vi "Compute Chirp Parameters-Core.vi"(10 "AOL_Globals":T3={"Imaging Protocol"=enum."AOL Z-Stack", "Number of POI"=0, "Number of Miniscans"=0, "Number of Trials"=0, "Number of Cycles "=0, "# Averaged Frames"=0, "Laser power (%)"=0, "Pockels (V)"=0.0, "Acquisition Length (sec)"=0.0, "Fill time (us)"=0.0, "POI Dwell time (us)"=0.0, "Miniscan Dwell time per pixel (us)"=0.0, "PMT 1"=0.0, "PMT 2"=0.0, "Back Apperture (mA)"=0.0, "Frame Size"=0, "Center Frequency"=0.0, "Field of View (um)"=175.0, "Field of View (norm)"=0.0, "DwellTime (us)"=0.0, "Ref Dwell Time (us)"=0.0, "Wavelength (nm)"=0.0, "Zoom"=0.0, "AOL Z"=0.0, "AOL Mode"=enum."Raster", "GridXY"=0.0, "GridZ"=0.0, "TriggerPeriod (sec)"=0.0, "Number of Pixels in Miniscan"=0, "Experiment folder path"=path "", "X centre"=0.0, "Y centre"=0.0, "Angle (degrees)"=0.0, "Angle Xs (degrees)"=0.0, "Angle Ys (degrees)"=0.0, "Plane Mode"=0, "Threshold"=[], "Regenerate Chirps"=FALSE, "Rectangle ROI length (pixels)"=0, "Rectangle ROI height (pixels)"=0, "AOD fill"=4900, "StartupDelay"=0, "Samples Wait after Trigger"=5080, "Slip Cycle"=600000, "Add Cycle"=TRUE, "Functional Mode"=enum."Point", "Z Start"=0.0, "Z Stop"=0.0, "# Planes"=0, "Total Pixels"=0, "Variable Miniscan Pixels"=[], "Use Variable Length"=FALSE, "Use Variable Resolution"=FALSE, "Laser power (%) at Z Start"=0, "Laser power (%) at Z Stop"=0, "Ref Z Step"=0} {"Angle Ys (degrees)" format="%#.6g"; "Angle Xs (degrees)" format="%#.6g"; "Plane Mode" items=["XY Plane", "XZ Plane", "YZ Plane", "arbitraryplane"]; "Frame Size" items=["100X100"=100, "128X128"=128, "200X200"=200, "256X256"=256, "512X512"=512, "1024x1024"=1024, "2048x2048"=2048]; "Back Apperture (mA)" format="%#.6g"; "Pockels (V)" format="%#.6g"; "PMT 2" format="%#.6g"; "PMT 1" format="%#.6g"; "Angle (degrees)" format="%#.6g"; "POI Dwell time (us)" format="%#.6g"}, 11 "Chirp in":cluster{"HexPackets":string[]}) -> (0 "error out":errorcluster, 1 "Z-stack chirp parameters":cluster{"HexPackets":string[]}[](array[cluster]), 2 "# of Z-planes":i32, 3 "Chirp out":cluster{"HexPackets":string[]})   [LabVIEW 2020]
uses:
  Typedefs/Controls/AOL_Globals.ctl
  Typedefs/Imaging Protocols enum.ctl
  Typedefs/Frame Size.ctl
  Typedefs/AOL modes.ctl
  Typedefs/Plane Mode.ctl
  Typedefs/Functional Mode.ctl
  Typedefs/ROI XY coordinates cluster.ctl
  Typedefs/Chirp_ABCD.ctl
  Typedefs/Read Write Enum.ctl
  Global Variables/General Globals.vi
panel:
  out "Chirp Parameters":T1
  out "ROI Coordinates (broken down to miniscans)":T2
  out "HexPackets":string[](array[string])
  out "AOL_Globals 2":T3={"Imaging Protocol"=enum."Live Imaging", "Number of POI"=0, "Number of Miniscans"=0, "Number of Trials"=0, "Number of Cycles "=0, "# Averaged Frames"=0, "Laser power (%)"=0, "Pockels (V)"=0.0, "Acquisition Length (sec)"=0.0, "Fill time (us)"=0.0, "POI Dwell time (us)"=0.0, "Miniscan Dwell time per pixel (us)"=0.0, "PMT 1"=0.0, "PMT 2"=0.0, "Back Apperture (mA)"=0.0, "Frame Size"=200, "Center Frequency"=0.0, "Field of View (um)"=175.0, "Field of View (norm)"=0.0, "DwellTime (us)"=0.0, "Ref Dwell Time (us)"=0.0, "Wavelength (nm)"=0.0, "Zoom"=0.0, "AOL Z"=0.0, "AOL Mode"=enum."Raster", "GridXY"=0.0, "GridZ"=0.0, "TriggerPeriod (sec)"=0.0, "Number of Pixels in Miniscan"=0, "Experiment folder path"=path "", "X centre"=0.0, "Y centre"=0.0, "Angle (degrees)"=0.0, "Angle Xs (degrees)"=0.0, "Angle Ys (degrees)"=0.0, "Plane Mode"=0, "Threshold"=[], "Regenerate Chirps"=FALSE, "Rectangle ROI length (pixels)"=0, "Rectangle ROI height (pixels)"=0, "AOD fill"=4900, "StartupDelay"=0, "Samples Wait after Trigger"=5080, "Slip Cycle"=600000, "Add Cycle"=TRUE, "Functional Mode"=enum."Point", "Z Start"=0.0, "Z Stop"=0.0, "# Planes"=0, "Total Pixels"=0, "Variable Miniscan Pixels"=[], "Use Variable Length"=FALSE, "Use Variable Resolution"=FALSE, "Laser power (%) at Z Start"=0, "Laser power (%) at Z Stop"=0, "Ref Z Step"=0} {"Angle Ys (degrees)" format="%#.6g"; "Angle Xs (degrees)" format="%#.6g"; "Plane Mode" items=["XY Plane", "XZ Plane", "YZ Plane", "arbitraryplane"]; "Frame Size" items=["100X100"=100, "128X128"=128, "200X200"=200, "256X256"=256, "512X512"=512, "1024x1024"=1024, "2048x2048"=2048]; "Back Apperture (mA)" format="%#.6g"; "Pockels (V)" format="%#.6g"; "PMT 2" format="%#.6g"; "PMT 1" format="%#.6g"; "Angle (degrees)" format="%#.6g"; "POI Dwell time (us)" format="%#.6g"}
  out "?":i32
  out "?":i32
  out "Execution time 2":u32
  out "Execution time":u32
  out "Imaging Protocol":T4
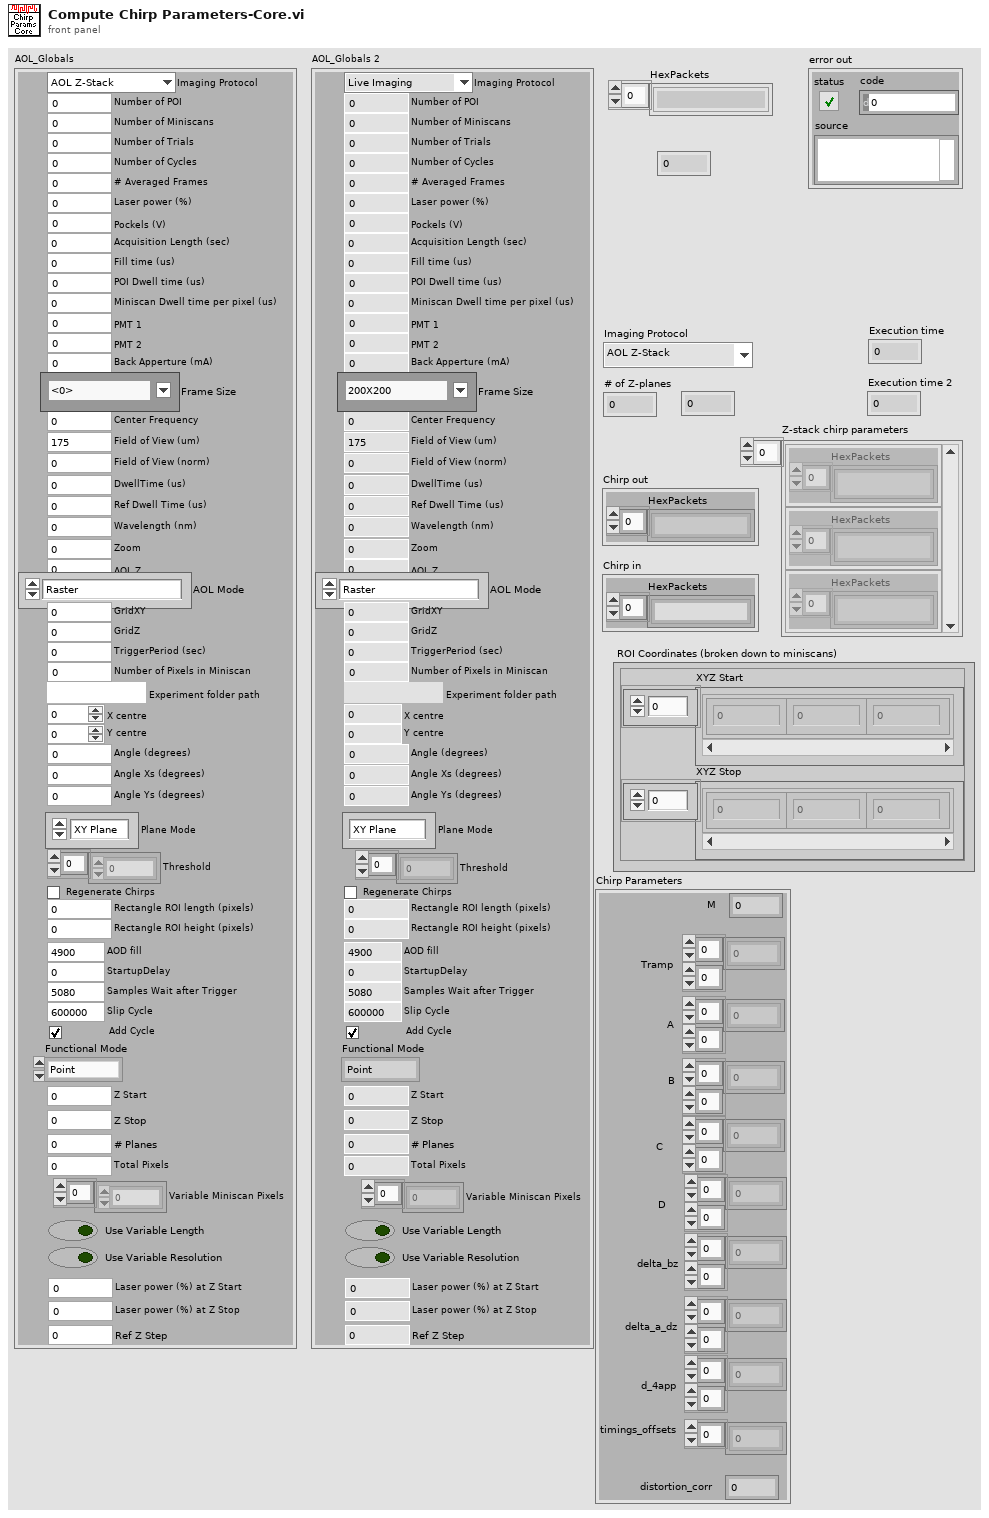
[diagram p1: front panel]
types:
  T1 = typedef "Chirp_ABCD.ctl" = cluster{"M ":dbl, "Tramp":dbl[][], "A":dbl[][], "B":dbl[][], "C":dbl[][], "D":dbl[][], "delta_bz":dbl[][], "delta_a_dz":dbl[][], "d_4app":dbl[][], "timings_offsets":dbl[], "distortion_corr":dbl}
  T2 = typedef "ROI XY coordinates cluster.ctl" = cluster{"XYZ Start":cluster{"X":sgl, "Y":sgl, "Z":sgl}[], "XYZ Stop":cluster{"X":sgl, "Y":sgl, "Z":sgl}[]}
  T3 = typedef "AOL_Globals.ctl" = cluster{"Imaging Protocol":T4, "Number of POI":u16, "Number of Miniscans":u16, "Number of Trials":u16, "Number of Cycles ":u64, "# Averaged Frames":u16, "Laser power (%)":u8, "Pockels (V)":dbl, "Acquisition Length (sec)":dbl, "Fill time (us)":dbl, "POI Dwell time (us)":dbl, "Miniscan Dwell time per pixel (us)":dbl, "PMT 1":dbl, "PMT 2":dbl, "Back Apperture (mA)":dbl, "Frame Size":T5, "Center Frequency":dbl, "Field of View (um)":dbl, "Field of View (norm)":dbl, "DwellTime (us)":dbl, "Ref Dwell Time (us)":dbl, "Wavelength (nm)":dbl, "Zoom":dbl, "AOL Z":dbl, "AOL Mode":T6, "GridXY":dbl, "GridZ":dbl, "TriggerPeriod (sec)":dbl, "Number of Pixels in Miniscan":u16, "Experiment folder path":path, "X centre":dbl, "Y centre":dbl, "Angle (degrees)":dbl, "Angle Xs (degrees)":dbl, "Angle Ys (degrees)":dbl, "Plane Mode":T7, "Threshold":u16[], "Regenerate Chirps":bool, "Rectangle ROI length (pixels)":u16, "Rectangle ROI height (pixels)":u16, "AOD fill":u16, "StartupDelay":i32, "Samples Wait after Trigger":u16, "Slip Cycle":u32, "Add Cycle":bool, "Functional Mode":T8, "Z Start":dbl, "Z Stop":dbl, "# Planes":i32, "Total Pixels":i32, "Variable Miniscan Pixels":u16[], "Use Variable Length":bool, "Use Variable Resolution":bool, "Laser power (%) at Z Start":u8, "Laser power (%) at Z Stop":u8, "Ref Z Step":i8}
  T4 = typedef "Imaging Protocols enum.ctl" = enum16{"AOL Z-Stack", "Motor Z Stack", "Parameter Sweep", "Functional Acquisition", "Single Plane Acquisition", "Volume Acquisition", "Live Imaging", "Live Plane Imaging", "Live Volume Imaging"}
  T5 = typedef "Frame Size.ctl" = u16
  T6 = typedef "AOL modes.ctl" = enum16{"Raster", "Structural", "Pointing", "Mini Scan", "Alignment"}
  T7 = typedef "Plane Mode.ctl" = u16
  T8 = typedef "Functional Mode.ctl" = enum16{"Point", "Line", "Patch", "Plane", "Volume"}
  T9 = typedef "Read Write Enum.ctl" = enum16{"Read", "Write"}
  T10 = cluster{"XYZ Start":cluster{"X":sgl, "Y":sgl, "Z":sgl}[], "XYZ Stop":cluster{"X":sgl, "Y":sgl, "Z":sgl}[]}
  T11 = typedef "ROI parameters data type.ctl" = cluster{"ROI index":dbl, "ROI ID":dbl, "ROI Time (ns)":dbl, "Pixels in ROI":dbl, "X start":dbl, "Y start":dbl, "Z start":dbl, "X stop":dbl, "Y stop":dbl, "Z stop":dbl, "Angle (deg)":dbl, "Composite ID":dbl, "Number of lines":dbl, "Frame Size":dbl, "Zoom":dbl, "Laser Power (%)":dbl, "ROI group ID":dbl, "Resolution":dbl, "Dwell Time per pixel":dbl, "Pixels per miniscan":dbl, "Original FOV (um)":dbl, "Apparent Frame Size":dbl, "Z Plane Idx":i32[], "Z Plane codes":i32[]}
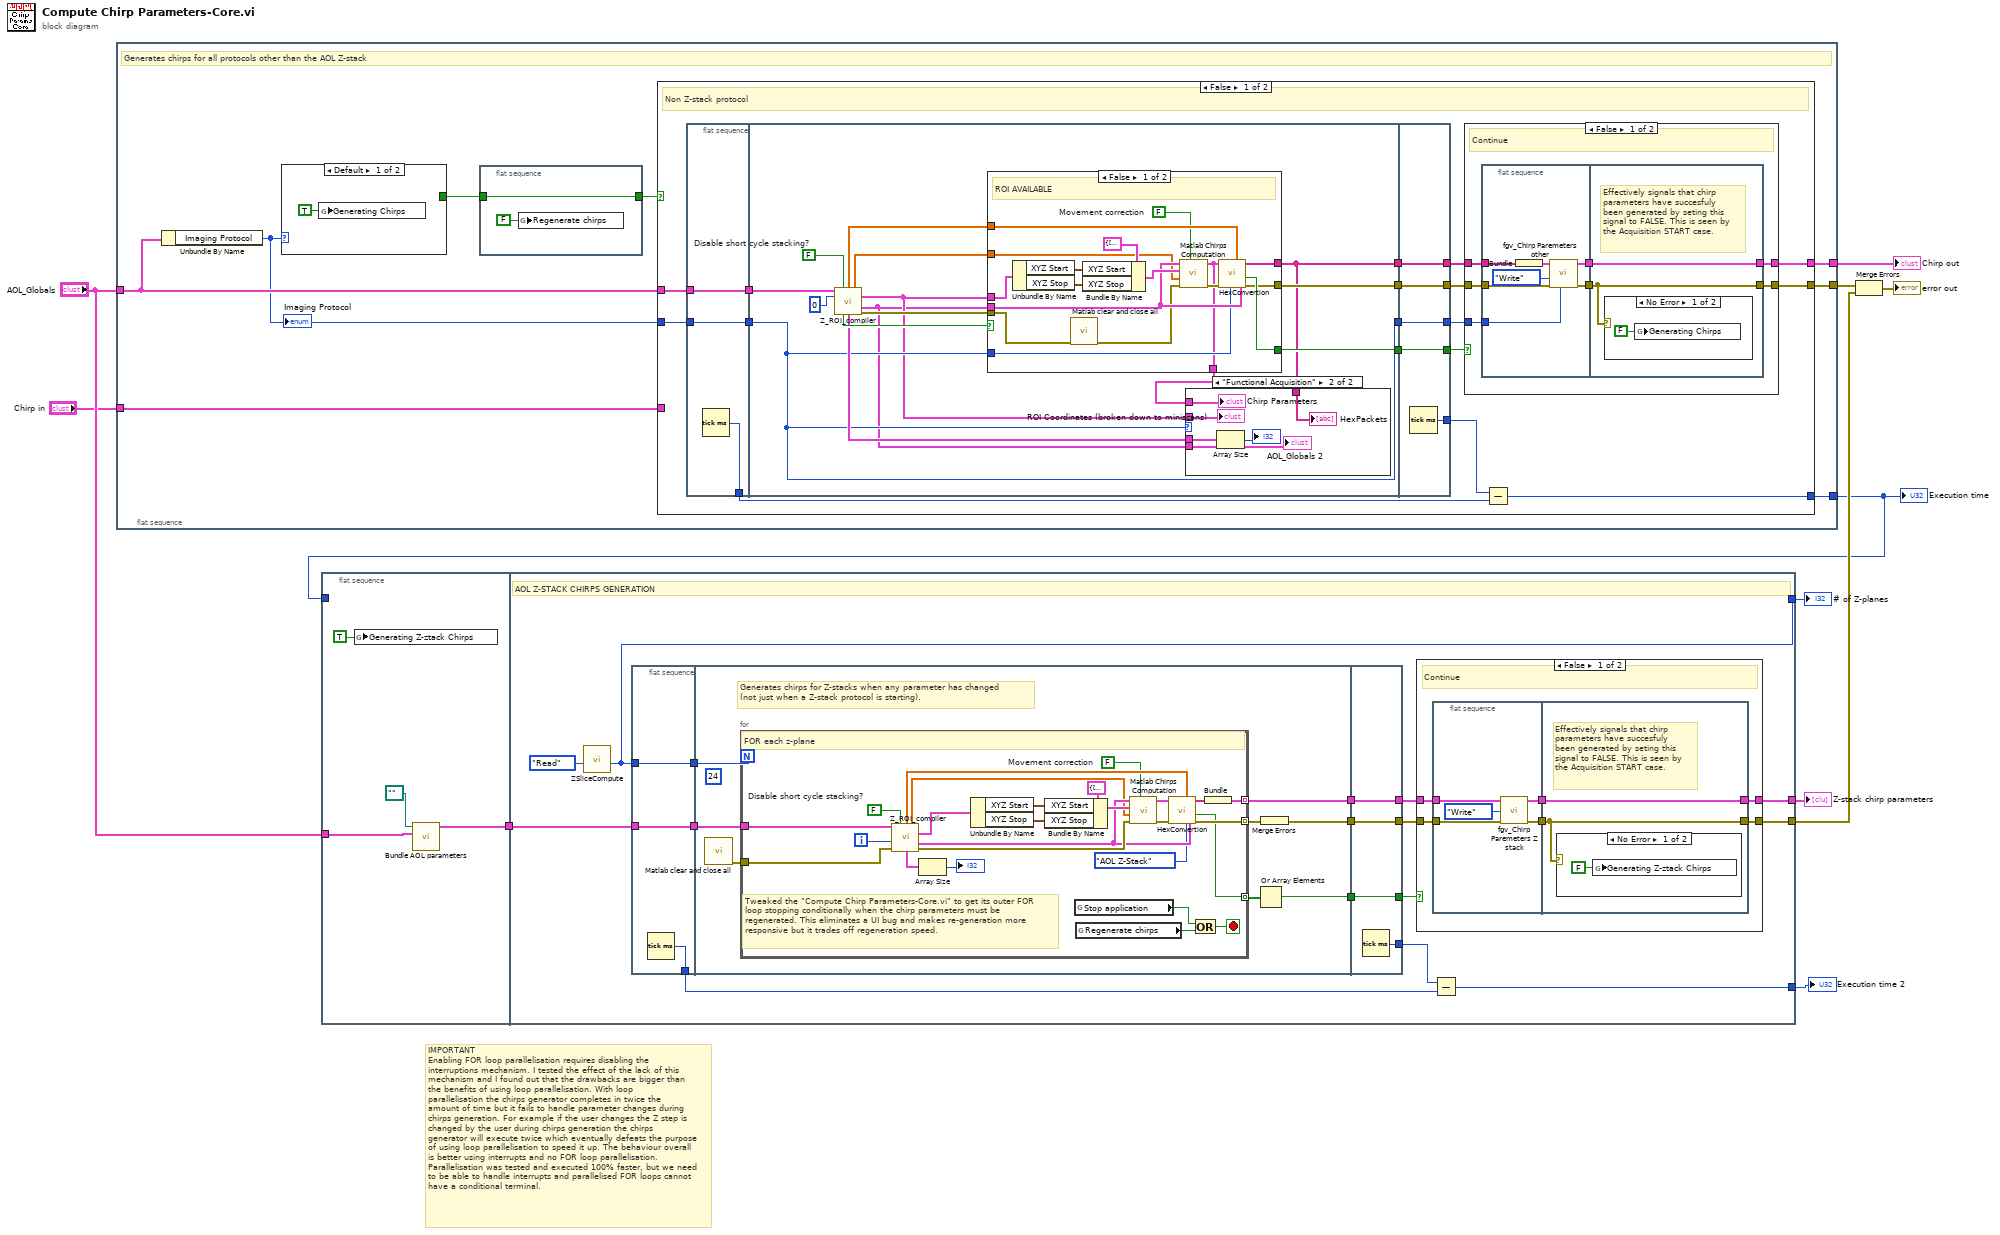
[diagram p0: block diagram]
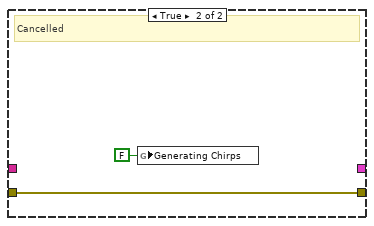
[diagram p5: hidden frame]
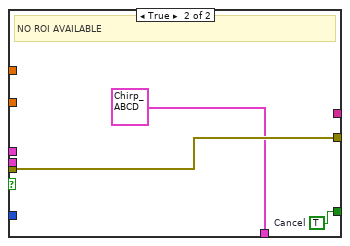
[diagram p7: hidden frame]
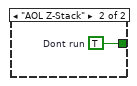
[diagram p9: hidden frame]
diagram:
  # "IMPORTANT\nEnabling FOR loop parallelisation requires disabling the interruptions mechanism. I tested the effect of the lack of this mechanism and I found out that the drawbacks are bigger than the benefits of using loop parallelisation. With loop parallelisation the chirps generator completes in twice the amount of time but it fails to handle parameter changes during chirps generation. For example if the user changes the Z step is changed by the user during chirps generation the chirps generator will execute twice which eventually defeats the purpose of using loop parallelisation to speed it up. The behaviour overall is better using interrupts and no FOR loop parallelisation. Parallelisation was tested and executed 100% faster, but we need to be able to handle interrupts and parallelised FOR loops cannot have a conditional terminal."
  n1 = flat-sequence {
    tunnel: [w19] -> w7
    tunnel: [w18] -> w2
    tunnel: [w17] -> w1
    tunnel: "AOL_Globals" -> [w16]
    tunnel: "Chirp in" -> [w15]
    frame #0 {
      # "Generates chirps for all protocols other than the AOL Z-stack"
      n2 = Unbundle By Name(w16) -> ("Imaging Protocol"=w12:T4)
      "Imaging Protocol" <- w12
      n3 = case shown="Default" w12 {
        tunnel: [_ w109] -> w14
        frame Default {
          n4 = global write "General Globals.vi" "Generating Chirps"(TRUE ("Generating Chirps")) -> ()
        }
        frame "AOL Z-Stack" {
          w109 = TRUE  # Dont run
        }
      }
      n5 = flat-sequence {
        tunnel: w14 -> [w20]
        tunnel: [w20] -> w13
        frame #0 {
          n6 = global write "General Globals.vi" "Regenerate chirps"(FALSE ("Regenerate chirps")) -> ()
        }
      }
      n7 = case shown="False" w13 {
        tunnel: [w38 w107] -> w19
        tunnel: [w37 _] -> w18
        tunnel: [w36 _] -> w17
        tunnel: w16 -> [w35 _]
        tunnel: w15 -> [_ w107]
        tunnel: w12 -> [w25 _]
        frame False {
          # "Non Z-stack protocol"
          n8 = flat-sequence {
            tunnel: w35 -> [w60]
            tunnel: [w60] -> w34
            tunnel: [w59] -> w29
            tunnel: w25 -> [w58]
            tunnel: [w58] -> w22
            tunnel: [w66] -> w33
            tunnel: [w74] -> w32
            tunnel: w34 -> [w67]
            tunnel: [w75] -> w31
            tunnel: [w65] -> w23
            tunnel: w22 -> [w65]
            tunnel: [w105] -> w27
            tunnel: [w106] -> w28
            tunnel: w33 -> [w106]
            tunnel: w32 -> [w105]
            tunnel: [w104] -> w30
            tunnel: [w103] -> w26
            tunnel: w31 -> [w103]
            tunnel: [w102] -> w24
            tunnel: w23 -> [w102]
            frame #0 {
              n9 = Tick Count (ms)() -> (millisecond timer value=w59:u32)
            }
            frame #1 {
              w69 = FALSE  # Disable short cycle stacking?
              n10 = call "Z_ROI_compiler.vi"("AOL_Globals"=w67, "dISABLE"=w69, "Acquired z-plane index / volume index"=0) -> ("Laser(V)"=w63:dbl[], "Zoom"=w71:dbl[], "ROI Coordinates (broken down to miniscans)"=w64:T2, "AOL_Globals"=w61:T3, "NO ROI AVAILABLE!!!"=w70:bool, "ROI Attributes (broken down to miniscans)"=w68:T11[], "error out"=w72:errorcluster)  [unwired: 5 in, 1 out]
              n11 = case shown="False" w70 {
                tunnel: w64 -> [w98 _]
                tunnel: w72 -> [w86 w101]
                tunnel: w61 -> [w92 _]
                tunnel: w71 -> [w91 _]
                tunnel: [w90 _] -> w66
                tunnel: [w89 w100] -> w75
                tunnel: [w88 w101] -> w74
                tunnel: w65 -> [w87 _]
                tunnel: w63 -> [w84 _]
                tunnel: [w82 T1 {"M "=0.0, "Tramp"=[], "A"=[], "B"=[], "C"=[], "D"=[], "delta_bz"=[], "delta_a_dz"=[], "d_4app"=[], "timings_offsets"=[], "distortion_corr"=0.0} ("Chirp Parameters")] -> w62
                frame False {
                  w83 = FALSE  # Movement correction
                  # "ROI AVAILABLE"
                  n12 = Unbundle By Name(w98) -> ("XYZ Start"=w95:cluster{"X":sgl, "Y":sgl, "Z":sgl}[], "XYZ Stop"=w94:cluster{"X":sgl, "Y":sgl, "Z":sgl}[])
                  n13 = call "Matlab clear and close all.vi"("error in (no error)"=w86) -> ("error out"=w85:errorcluster)  [unwired: 10 in]
                  n14 = Bundle By Name(cluster=T10 {"XYZ Start"=[{"X"=0.0, "Y"=0.0, "Z"=0.0}], "XYZ Stop"=[]} ("ROI Coordinates"), "XYZ Start"=w95, "XYZ Stop"=w94) -> (w97:T10)
                  n15 = call "Matlab Chirps Computation.vi"("Movement correction"=w83, "error in"=w85, "Zoom"=w91, "ROI Coordinates"=w97, "AOL_Globals"=w92) -> ("error out"=w93:errorcluster, "Chirp Parameters"=w82:T1)  [unwired: 3 in, 2 out]
                  n16 = call "HexConvertion.vi"("Imaging Protocol"=w87, "Laser(V)"=w84, "AOL_Globals"=w92, "error in (no error)"=w93, "Chirp Parameters"=w82) -> ("error out"=w88:errorcluster, "Interrupted"=w89:bool, "HexPackets"=w90:string[])  [unwired: 4 in]
                }
                frame True {
                  w100 = TRUE  # Cancel
                  # "NO ROI AVAILABLE"
                }
              }
              n17 = case shown="\"Functional Acquisition\"" w65 {
                tunnel: w68 -> [_ w80]
                tunnel: w61 -> [_ w79]
                tunnel: w66 -> [_ w78]
                tunnel: w64 -> [_ w77]
                tunnel: w62 -> [_ w76]
                frame Default {
                }
                frame "Functional Acquisition" {
                  n18 = Array Size(array=w80) -> (size(s)=→"?":i32)
                  "AOL_Globals 2" <- w79
                  "HexPackets" <- w78
                  "ROI Coordinates (broken down to miniscans)" <- w77
                  "Chirp Parameters" <- w76
                }
              }
            }
            frame #2 {
              n19 = Tick Count (ms)() -> (millisecond timer value=w104:u32)
            }
          }
          n20 = case shown="False" w26 {
            tunnel: [w45 _] -> w38
            tunnel: w28 -> [w44 _]
            tunnel: [w43 w57] -> w37
            tunnel: w27 -> [w42 w57]
            tunnel: w24 -> [w39 _]
            frame False {
              # "Continue"
              n21 = flat-sequence {
                tunnel: w44 -> [w52]
                tunnel: w42 -> [w49]
                tunnel: [w47] -> w41
                tunnel: [w48] -> w40
                tunnel: w39 -> [w46]
                tunnel: [w53] -> w43
                tunnel: [w54] -> w45
                tunnel: w41 -> [w54]
                tunnel: w40 -> [w53]
                frame #0 {
                  n22 = Bundle("HexPackets"=w52) -> (w51:cluster{"HexPackets":string[]})  [unwired: 1 in]
                  n23 = call "fgv_Chirp Paremeters other.vi"("Imaging Protocol in"=w46, "error in"=w49, "Function"=Read_Write_Enum."Write", "Chirps in"=w51) -> ("error out"=w48:errorcluster, "Chirps"=w47:cluster{"HexPackets":string[]})  [unwired: 5 in, 1 out]
                }
                frame #1 {
                  # "Effectively signals that chirp parameters have succesfuly been generated by seting this signal to FALSE. This is seen by the Acquisition START case."
                  n24 = case shown="No Error" w53 {
                    frame No Error {
                      n25 = global write "General Globals.vi" "Generating Chirps"(FALSE ("Generating Chirps")) -> ()
                    }
                    frame Error {
                    }
                  }
                }
              }
            }
            frame True {
              # "Cancelled"
              n26 = global write "General Globals.vi" "Generating Chirps"(FALSE ("Generating Chirps")) -> ()
            }
          }
          n27 = Subtract(x=w30, y=w29) -> (x-y=w36:u32)
        }
        frame True {
          # "Z-stack protocol"
        }
      }
    }
  }
  n28 = flat-sequence {
    tunnel: "AOL_Globals" -> [w113]
    tunnel: [w112] -> w11
    tunnel: [w110] -> _
    tunnel: w1 -> [w110]
    tunnel: w11 -> [w126]
    tunnel: [w130] -> w8
    tunnel: [w129] -> w3
    tunnel: [w128] -> w5
    tunnel: [w127] -> w9
    frame #0 {
      n29 = global write "General Globals.vi" "Generating Z-ztack Chirps"(TRUE ("Generating Chirps")) -> ()
      n30 = call "Bundle AOL parameters.vi"("AOL_Globals in"=w113, "Experiment folder path"=path "") -> ("AOL_Globals out"=w112:T3)  [unwired: 9 in]
    }
    frame #1 {
      # "AOL Z-STACK CHIRPS GENERATION"
      n31 = call "ZSliceCompute.vi"("Function"=Read_Write_Enum."Read") -> ("# of Z-planes"=w128:i32)  [unwired: 7 in, 3 out]
      n32 = flat-sequence {
        tunnel: w128 -> [w147]
        tunnel: w126 -> [w148]
        tunnel: [w148] -> w125
        tunnel: [w147] -> w124
        tunnel: [w146] -> w119
        tunnel: [w150] -> w123
        tunnel: [w154] -> w122
        tunnel: w125 -> [w156]
        tunnel: w124 -> [w153]
        tunnel: [w151] -> w121
        tunnel: [w185] -> w117
        tunnel: [w186] -> w118
        tunnel: w123 -> [w186]
        tunnel: w122 -> [w185]
        tunnel: [w184] -> w120
        tunnel: [w183] -> w116
        tunnel: w121 -> [w183]
        frame #0 {
          n33 = Tick Count (ms)() -> (millisecond timer value=w146:u32)
        }
        frame #1 {
          (unwired) 24
          # "Generates chirps for Z-stacks when any parameter has changed\n(not just when a Z-stack protocol is starting)."
          n34 = call "Matlab clear and close all.vi"() -> ("error out"=w149:errorcluster)  [unwired: 11 in]
          n35 = for {
            N: w153 -> [_]
            tunnel: [w182] -> w155 mode=indexing
            tunnel: [w181] -> w150 mode=indexing
            tunnel: w156 -> [w180]
            tunnel: [w178] -> w152 mode=indexing
            tunnel: w149 -> [w174]
            i -> [w179]
            stop <- w175 stop-if-true
            w157 = FALSE  # Movement correction
            w162 = FALSE  # Disable short cycle stacking?
            # "Tweaked the \"Compute Chirp Parameters-Core.vi\" to get its outer FOR loop stopping conditionally when the chirp parameters must be regenerated. This eliminates a UI bug and makes re-generation more responsive but it trades off regeneration speed."
            # "FOR each z-plane"
            n36 = call "Z_ROI_compiler.vi"("AOL_Globals"=w180, "dISABLE"=w162, "Acquired z-plane index / volume index"=w179, "error in (no error)"=w174) -> ("Laser(V)"=w158:dbl[], "Zoom"=w163:dbl[], "ROI Coordinates (broken down to miniscans)"=w164:T2, "AOL_Globals"=w165:T3, "ROI Attributes (broken down to miniscans)"=w161:T11[], "error out"=w166:errorcluster)  [unwired: 4 in, 2 out]
            n37 = Array Size(array=w161) -> (size(s)=→"?":i32)
            n38 = Unbundle By Name(w164) -> ("XYZ Start"=w170:cluster{"X":sgl, "Y":sgl, "Z":sgl}[], "XYZ Stop"=w169:cluster{"X":sgl, "Y":sgl, "Z":sgl}[])
            n39 = Bundle By Name(cluster=T10 {"XYZ Start"=[{"X"=0.0, "Y"=0.0, "Z"=0.0}], "XYZ Stop"=[]} ("ROI Coordinates"), "XYZ Start"=w170, "XYZ Stop"=w169) -> (w172:T10)
            n40 = global read "General Globals.vi" "Stop application"() -> (w176:bool)
            n41 = global read "General Globals.vi" "Regenerate chirps"() -> (w177:bool)
            n42 = call "Matlab Chirps Computation.vi"("Movement correction"=w157, "error in"=w166, "Zoom"=w163, "ROI Coordinates"=w172, "AOL_Globals"=w165) -> ("error out"=w167:errorcluster, "Chirp Parameters"=w168:T1)  [unwired: 3 in, 2 out]
            n43 = call "HexConvertion.vi"("Imaging Protocol"=Imaging_Protocols_enum."AOL Z-Stack", "Laser(V)"=w158, "AOL_Globals"=w165, "error in (no error)"=w167, "Chirp Parameters"=w168) -> ("error out"=w182:errorcluster, "Interrupted"=w178:bool, "HexPackets"=w173:string[])  [unwired: 4 in]
            n44 = Compound Arithmetic op=OR(w176, w177) -> (w175:bool)
            n45 = Bundle("HexPackets"=w173) -> (w181:cluster{"HexPackets":string[]})  [unwired: 1 in]
          }
          n46 = Or Array Elements(Boolean array=w152) -> (logical OR=w151:bool)
          n47 = Merge Errors(w155) -> (w154:errorcluster)
        }
        frame #2 {
          n48 = Tick Count (ms)() -> (millisecond timer value=w184:u32)
        }
      }
      n49 = case shown="False" w116 {
        tunnel: [w136 _] -> w130
        tunnel: w118 -> [w135 _]
        tunnel: [w134 w145] -> w129
        tunnel: w117 -> [w133 w145]
        frame False {
          # "Continue"
          n50 = flat-sequence {
            tunnel: w135 -> [w139]
            tunnel: w133 -> [w137]
            tunnel: [w140] -> w132
            tunnel: [w138] -> w131
            tunnel: [w142] -> w134
            tunnel: [w143] -> w136
            tunnel: w132 -> [w143]
            tunnel: w131 -> [w142]
            frame #0 {
              n51 = call "fgv_Chirp Paremeters Z stack.vi"("error in"=w137, "Function"=Read_Write_Enum."Write", "Z-stack Chirp parameters (all Z planes) in"=w139) -> ("error out"=w138:errorcluster, "Z-stack Chirp parameters (all Z planes)"=w140:cluster{"HexPackets":string[]}[])  [unwired: 7 in]
            }
            frame #1 {
              # "Effectively signals that chirp parameters have succesfuly been generated by seting this signal to FALSE. This is seen by the Acquisition START case."
              n52 = case shown="No Error" w142 {
                frame No Error {
                  n53 = global write "General Globals.vi" "Generating Z-ztack Chirps"(FALSE ("Generating Chirps")) -> ()
                }
                frame Error {
                }
              }
            }
          }
        }
        frame True {
          # "Cancelled"
        }
      }
      n54 = Subtract(x=w120, y=w119) -> (x-y=w127:u32)
    }
  }
  n55 = Merge Errors(w2, w3) -> (→"error out":errorcluster)
  "Z-stack chirp parameters" <- w8
  "# of Z-planes" <- w5
  "Execution time" <- w1
  "Execution time 2" <- w9
  "Chirp out" <- w7
